vi "Teardown.vi"(8 "error in (no error)":errorcluster, 11 "Teardown Error Test Dummy In":refnum<class "Teardown Error Test Dummy.lvclass">) -> (0 "error out":errorcluster, 3 "Teardown Error Test Dummy Out":refnum<class "Teardown Error Test Dummy.lvclass">)   [LabVIEW 2020, in "Teardown Error Test Dummy.lvclass"]
doc: "Setup method called by the testing framework before each test method is called."
uses:
  Teardown Error Test Dummy.lvclass
  Teardown Error Test Dummy.lvclass/Teardown Error Test Dummy.ctl
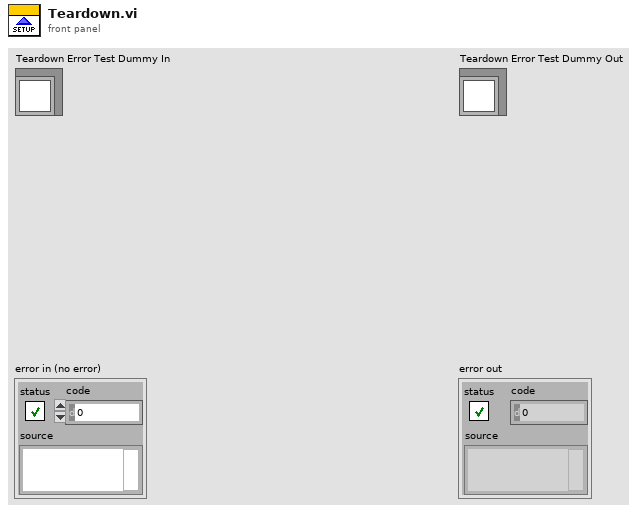
[diagram p1: front panel]
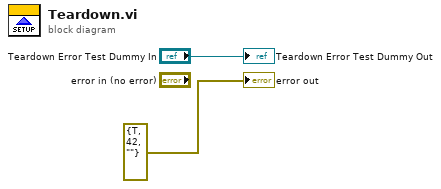
[diagram p0: block diagram]
diagram:
  "error out" <- errorcluster {"status"=TRUE, "code"=42, "source"=""} ("error out")
  "Teardown Error Test Dummy Out" <- "Teardown Error Test Dummy In"
